vi "Position Check.vi"() -> ()   [LabVIEW 2024]
panel:
  out "end":u32
  out "End pos":u32
  out "Start pos":u32
  in  "End off":u32
  out "x .and. y?":u32
  out "start":u32
  in  "Start off":u32
  in  "Trig pos":u32
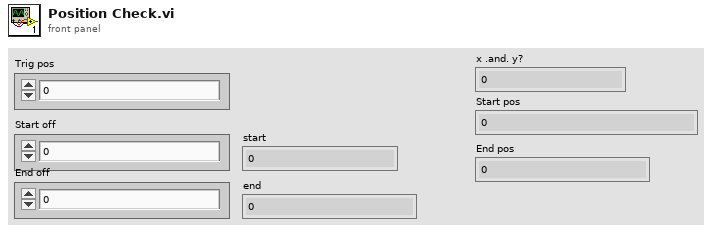
[diagram p1: front panel]
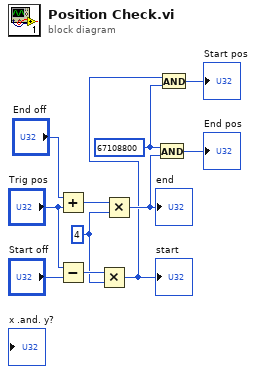
[diagram p0: block diagram]
diagram:
  w2 = u32 4 ("y")
  w6 = u32 67108800 ("y")
  n1 = Add(x="End off", y="Trig pos") -> (x+y=w8:u32)
  n2 = Subtract(x="Trig pos", y="Start off") -> (x-y=w3:u32)
  n3 = Multiply(x=w3, y=w2) -> (x*y=w1:u32)
  "start" <- w1
  n4 = Multiply(x=w8, y=w2) -> (x*y=w7:u32)
  "end" <- w7
  n5 = And(x=w6, y=w7) -> (x .and. y?=→"End pos":u32)
  n6 = And(x=w1, y=w6) -> (x .and. y?=→"Start pos":u32)
